vi "Emballage_BDD_correspondance_Code_barre_plusieurPossible.vi"(7 "tableau des codes barres":string[](array[string]), 8 "entrée d'erreur\n (pas d'erreur)":errorcluster caption="entrée d'erreur (pas d'erreur)", 9 "tableau des produits code FAS":string[](array[string]), 10 "Etiquette scanné":string, 11 "MulticolumnListbox en entrée":refnum<vi>) -> (0 "sortie d'erreur":errorcluster, 1 "index_produit":i32, 2 "message":string, 3 "Produit Code FAS":string)   [LabVIEW 2020]
uses:
  Modules/FS/60_FS_Controles/60_FS_SetGet.ctl
panel:
  out "Tableau_indice":i32[](array[numeric])
  out "sous-chaîne_6":string
  out "sous-chaîne_8":string
  out "sous-chaîne_9":string
  out "sous-chaîne_10":string
  out "sous-chaîne_11":string
  out "sous-chaîne_12":string
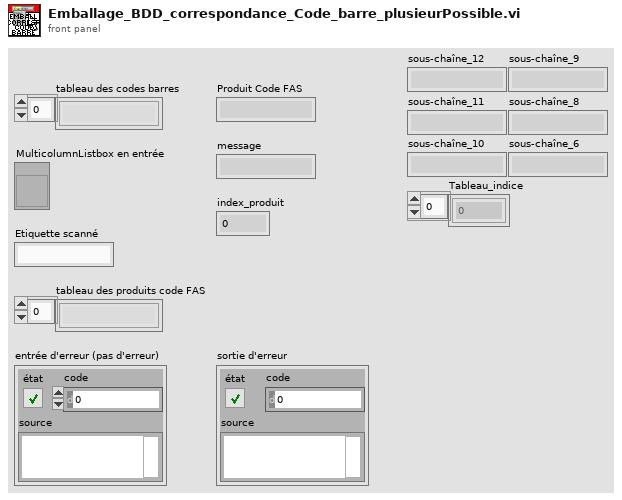
[diagram p1: front panel]
types:
  T1 = typedef "60_FS_SetGet.ctl" = enum16{"set", "get"}
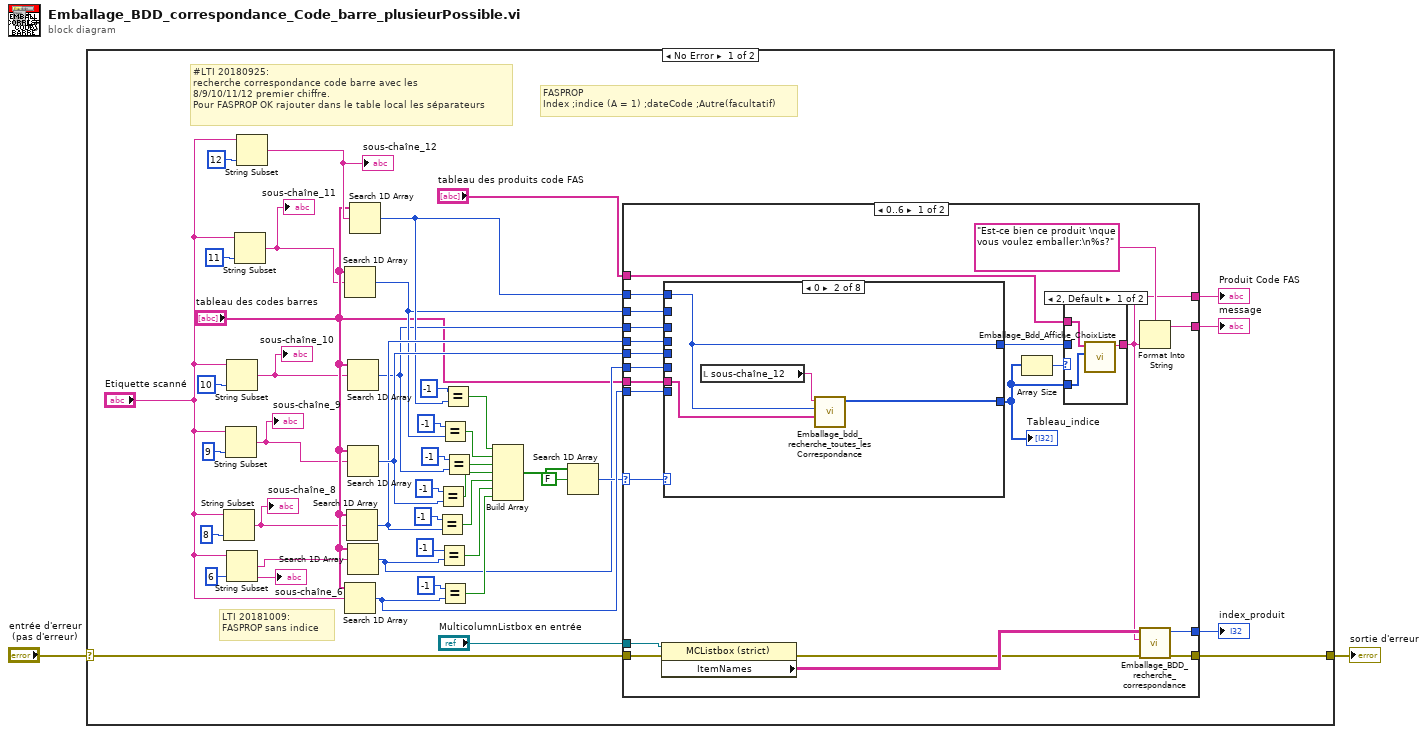
[diagram p0: block diagram]
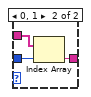
[diagram p2: hidden frame]
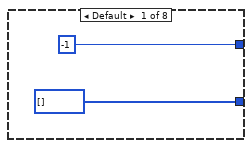
[diagram p3: hidden frame]
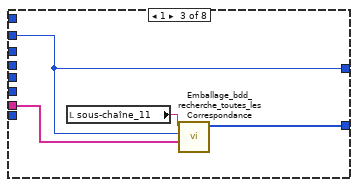
[diagram p4: hidden frame]
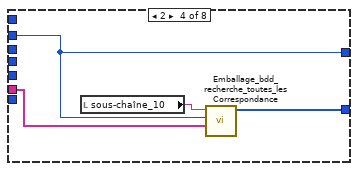
[diagram p5: hidden frame]
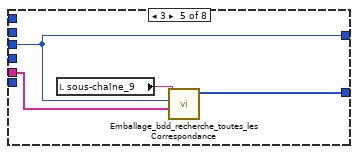
[diagram p6: hidden frame]
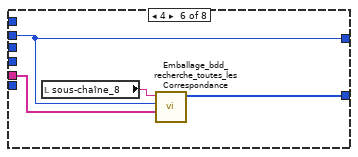
[diagram p7: hidden frame]
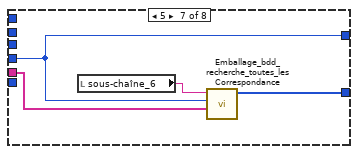
[diagram p8: hidden frame]
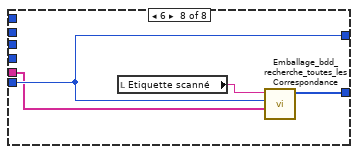
[diagram p9: hidden frame]
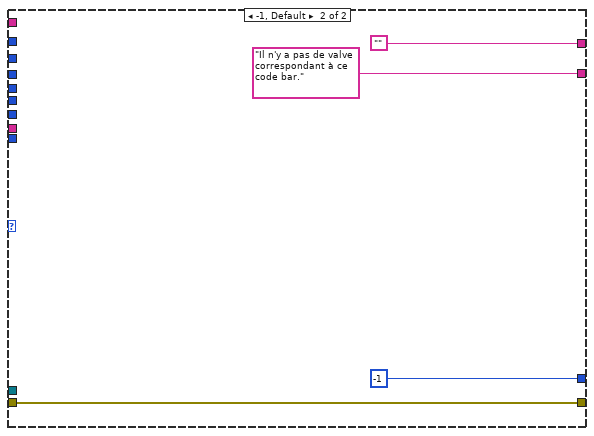
[diagram p10: hidden frame]
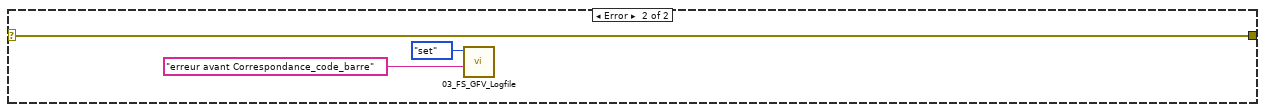
[diagram p11: hidden frame]
diagram:
  n1 = case shown="No Error" "entrée d'erreur\n (pas d'erreur)" {
    selector: "entrée d'erreur\n (pas d'erreur)" -> [w22 w112]
    tunnel: [w21 w112] -> w1
    frame No Error {
      # "LTI 20181009:\nFASPROP sans indice"
      # "#LTI 20180925:\nrecherche correspondance code barre avec les \n8/9/10/11/12 premier chiffre.\nPour FASPROP OK rajouter dans le table local les séparateurs"
      # "FASPROP\nIndex ;indice (A = 1) ;dateCode ;Autre(facultatif)"
      n2 = String Subset(string="Etiquette scanné", length (rest)=8 ("longueur (reste)")) -> (substring=w3:string)  [unwired: 1 in]
      "sous-chaîne_8" <- w3
      n3 = String Subset(string="Etiquette scanné", length (rest)=9 ("longueur (reste)")) -> (substring=w4:string)  [unwired: 1 in]
      "sous-chaîne_9" <- w4
      n4 = String Subset(string="Etiquette scanné", length (rest)=10 ("longueur (reste)")) -> (substring=w6:string)  [unwired: 1 in]
      "sous-chaîne_10" <- w6
      n5 = String Subset(string="Etiquette scanné", length (rest)=6 ("longueur (reste)")) -> (substring=w5:string)  [unwired: 1 in]
      "sous-chaîne_6" <- w5
      n6 = String Subset(string="Etiquette scanné", length (rest)=11 ("longueur (reste)")) -> (substring=w7:string)  [unwired: 1 in]
      "sous-chaîne_11" <- w7
      n7 = String Subset(string="Etiquette scanné", length (rest)=12 ("longueur (reste)")) -> (substring=w31:string)  [unwired: 1 in]
      "sous-chaîne_12" <- w31
      n8 = Search 1D Array(1D array="tableau des codes barres", element=w7) -> (index of element=w38:i32)  [unwired: 1 in]
      n9 = Search 1D Array(1D array="tableau des codes barres", element="Etiquette scanné") -> (index of element=w47:i32)  [unwired: 1 in]
      n10 = Search 1D Array(1D array="tableau des codes barres", element=w3) -> (index of element=w40:i32)  [unwired: 1 in]
      n11 = Search 1D Array(1D array="tableau des codes barres", element=w6) -> (index of element=w37:i32)  [unwired: 1 in]
      n12 = Search 1D Array(1D array="tableau des codes barres", element=w4) -> (index of element=w43:i32)  [unwired: 1 in]
      n13 = Search 1D Array(1D array="tableau des codes barres", element=w5) -> (index of element=w9:i32)  [unwired: 1 in]
      n14 = Search 1D Array(1D array="tableau des codes barres", element=w31) -> (index of element=w39:i32)  [unwired: 1 in]
      n15 = Equal?(x=-1, y=w40) -> (x = y?=w16:bool)
      n16 = Equal?(x=-1, y=w43) -> (x = y?=w17:bool)
      n17 = Equal?(x=-1, y=w9) -> (x = y?=w10:bool)
      n18 = Equal?(x=-1, y=w38) -> (x = y?=w19:bool)
      n19 = Equal?(x=-1, y=w47) -> (x = y?=w11:bool)
      n20 = Equal?(x=-1, y=w39) -> (x = y?=w20:bool)
      n21 = Equal?(x=-1, y=w37) -> (x = y?=w18:bool)
      n22 = Build Array(w20, w19, w18, w17, w16, w10, w11) -> (w29:bool[])
      n23 = Search 1D Array(1D array=w29, element=FALSE ("élément")) -> (index of element=w36:i32)  [unwired: 1 in]
      n24 = case shown="0..6" w36 {
        selector: w36 -> [w61 _]
        tunnel: "tableau des produits code FAS" -> [w69 _]
        tunnel: [w67 "Il n'y a pas de valve correspondant à ce code bar."] -> w25
        tunnel: [w64 ""] -> w45
        tunnel: w22 -> [w66 w107]
        tunnel: [w52 w107] -> w21
        tunnel: w37 -> [w59 _]
        tunnel: w38 -> [w58 _]
        tunnel: w39 -> [w57 _]
        tunnel: w40 -> [w56 _]
        tunnel: w43 -> [w55 _]
        tunnel: [w63 -1 ("élément")] -> w44
        tunnel: w47 -> [w54 _]
        tunnel: "MulticolumnListbox en entrée" -> [w62 _]
        tunnel: w9 -> [w51 _]
        tunnel: "tableau des codes barres" -> [w50 _]
        frame 0..6 {
          n25 = property on="Nœud de propriété" class="MCListbox (strict)"(reference=w62, error in=w66) -> (error out=w53:errorcluster, "ItemNames"=w65:string[][])  [unwired: 1 out]
          n26 = case shown="0" w61 {
            tunnel: [-1 ("index of element") w81 w83 w88 w92 w96 w100 w104] -> w60
            tunnel: w59 -> [_ _ _ w88 _ _ _ _]
            tunnel: w58 -> [_ _ w83 _ _ _ _ _]
            tunnel: w57 -> [_ w81 _ _ _ _ _ _]
            tunnel: w56 -> [_ _ _ _ _ w96 _ _]
            tunnel: w55 -> [_ _ _ _ w92 _ _ _]
            tunnel: w54 -> [_ _ _ _ _ _ _ w104]
            tunnel: w51 -> [_ _ _ _ _ _ w100 _]
            tunnel: w50 -> [_ w80 w82 w87 w91 w95 w99 w103]
            tunnel: [i32[] [] ("Tableau_Indice") w79 w84 w86 w90 w94 w98 w102] -> w48
            frame Default {
            }
            frame 0 {
              n27 = local read "sous-chaîne_12"() -> (w78:string)
              n28 = call "Emballage_bdd_recherche_toutes_les Correspondance.vi"("tableau des codes barres"=w80, "1er index"=w81, "Sous_chaine"=w78) -> ("Tableau_Indice"=w79:i32[])  [unwired: 8 in]
            }
            frame 1 {
              n29 = local read "sous-chaîne_11"() -> (w85:string)
              n30 = call "Emballage_bdd_recherche_toutes_les Correspondance.vi"("tableau des codes barres"=w82, "1er index"=w83, "Sous_chaine"=w85) -> ("Tableau_Indice"=w84:i32[])  [unwired: 8 in]
            }
            frame 2 {
              n31 = local read "sous-chaîne_10"() -> (w89:string)
              n32 = call "Emballage_bdd_recherche_toutes_les Correspondance.vi"("tableau des codes barres"=w87, "1er index"=w88, "Sous_chaine"=w89) -> ("Tableau_Indice"=w86:i32[])  [unwired: 8 in]
            }
            frame 3 {
              n33 = local read "sous-chaîne_9"() -> (w93:string)
              n34 = call "Emballage_bdd_recherche_toutes_les Correspondance.vi"("tableau des codes barres"=w91, "1er index"=w92, "Sous_chaine"=w93) -> ("Tableau_Indice"=w90:i32[])  [unwired: 8 in]
            }
            frame 4 {
              n35 = local read "sous-chaîne_8"() -> (w97:string)
              n36 = call "Emballage_bdd_recherche_toutes_les Correspondance.vi"("tableau des codes barres"=w95, "1er index"=w96, "Sous_chaine"=w97) -> ("Tableau_Indice"=w94:i32[])  [unwired: 8 in]
            }
            frame 5 {
              n37 = local read "sous-chaîne_6"() -> (w101:string)
              n38 = call "Emballage_bdd_recherche_toutes_les Correspondance.vi"("tableau des codes barres"=w99, "1er index"=w100, "Sous_chaine"=w101) -> ("Tableau_Indice"=w98:i32[])  [unwired: 8 in]
            }
            frame 6 {
              n39 = local read "Etiquette scanné"() -> (w105:string)
              n40 = call "Emballage_bdd_recherche_toutes_les Correspondance.vi"("tableau des codes barres"=w103, "1er index"=w104, "Sous_chaine"=w105) -> ("Tableau_Indice"=w102:i32[])  [unwired: 8 in]
            }
          }
          "Tableau_indice" <- w48
          n41 = Array Size(array=w48) -> (size(s)=w49:i32)
          n42 = case shown="2, Default" w49 {
            tunnel: w69 -> [w70 w75]
            tunnel: [w71 w74] -> w64
            tunnel: w60 -> [_ w73]
            tunnel: w48 -> [w72 _]
            frame 2, Default {
              n43 = call "Emballage_Bdd_Affiche_ChoixListe.vi"("Tableau_indice"=w72, "tableau des produits code FAS"=w70) -> ("Produit_code_FAS"=w71:string)  [unwired: 8 in, 1 out]
            }
            frame 0, 1 {
              n44 = Index Array(array=w75, index=w73) -> (element=w74:string)
            }
          }
          n45 = Format Into String(format string="Est-ce bien ce produit \nque vous voulez emballer:\n%s?", w64) -> (resulting string=w67:string)  [unwired: 2 in, 1 out]
          n46 = call "Emballage_BDD_recherche_correspondance.vi"("Error in"=w53, "Chaîne"=w64, "Tableau_IN"=w65) -> ("Error out"=w52:errorcluster, "élément"=w63:i32)  [unwired: 6 in, 1 out]
        }
        frame -1, Default {
        }
      }
      "Produit Code FAS" <- w45
      "index_produit" <- w44
      "message" <- w25
    }
    frame Error {
      n47 = call "03_FS_GFV_Logfile.vi"("Chaîne"="erreur avant Correspondance_code_barre", "States"=60_FS_SetGet."set") -> ()  [unwired: 8 in, 2 out]
    }
  }
  "sortie d'erreur" <- w1
